vi "GV_YscaleCursorInView.vi"(8 "error in (no error)":errorcluster, 11 "Gviewer in":refnum<class "Gviewer.lvclass">) -> (0 "error out":errorcluster, 3 "Gviewer out":refnum<class "Gviewer.lvclass">)   [LabVIEW 2020, in "Sgraph_lib_V1.lvlib" / "Gviewer.lvclass"]
doc: "Draw cursors and enable identification of a specific trace so it can be selected\nFor use with Y-scale move/delete action"
uses:
  Gviewer.lvclass
  Gviewer.lvclass/Gviewer.ctl
  b6d83b76-addd-4bb4-aca8-673370ce0a1b.vi
  <vilib>/Comparison/Equal/Equal Functor/Equal Functor.lvclass
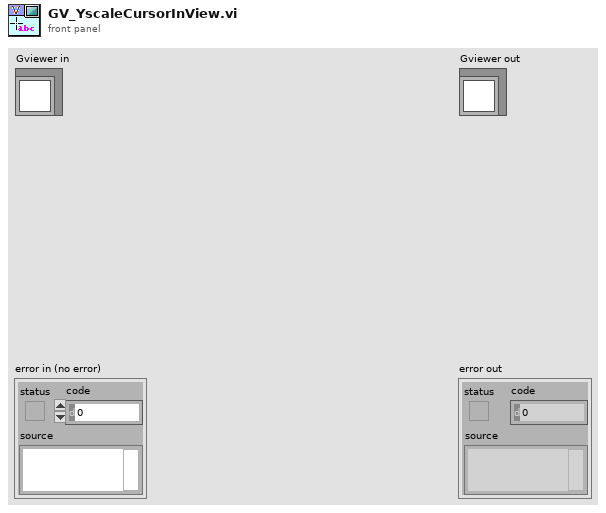
[diagram p1: front panel]
types:
  T1 = typedef "LVPoint32TypeDef.ctl" = cluster{"Horizontal":i32, "Vertical":i32}
  T2 = typedef "LVPositionTypeDef.ctl" = cluster{"Left":i32, "Top":i32}
  T3 = typedef "Sgraph_lib_V1.lvlib/Gviewer.lvclass/YgraphDef.ctl" = cluster{"Plot":i32, "X(%)":dbl}
  T4 = typedef "LVRectTypeDef.ctl" = cluster{"Left":i16, "Top":i16, "Right":i16, "Bottom":i16}
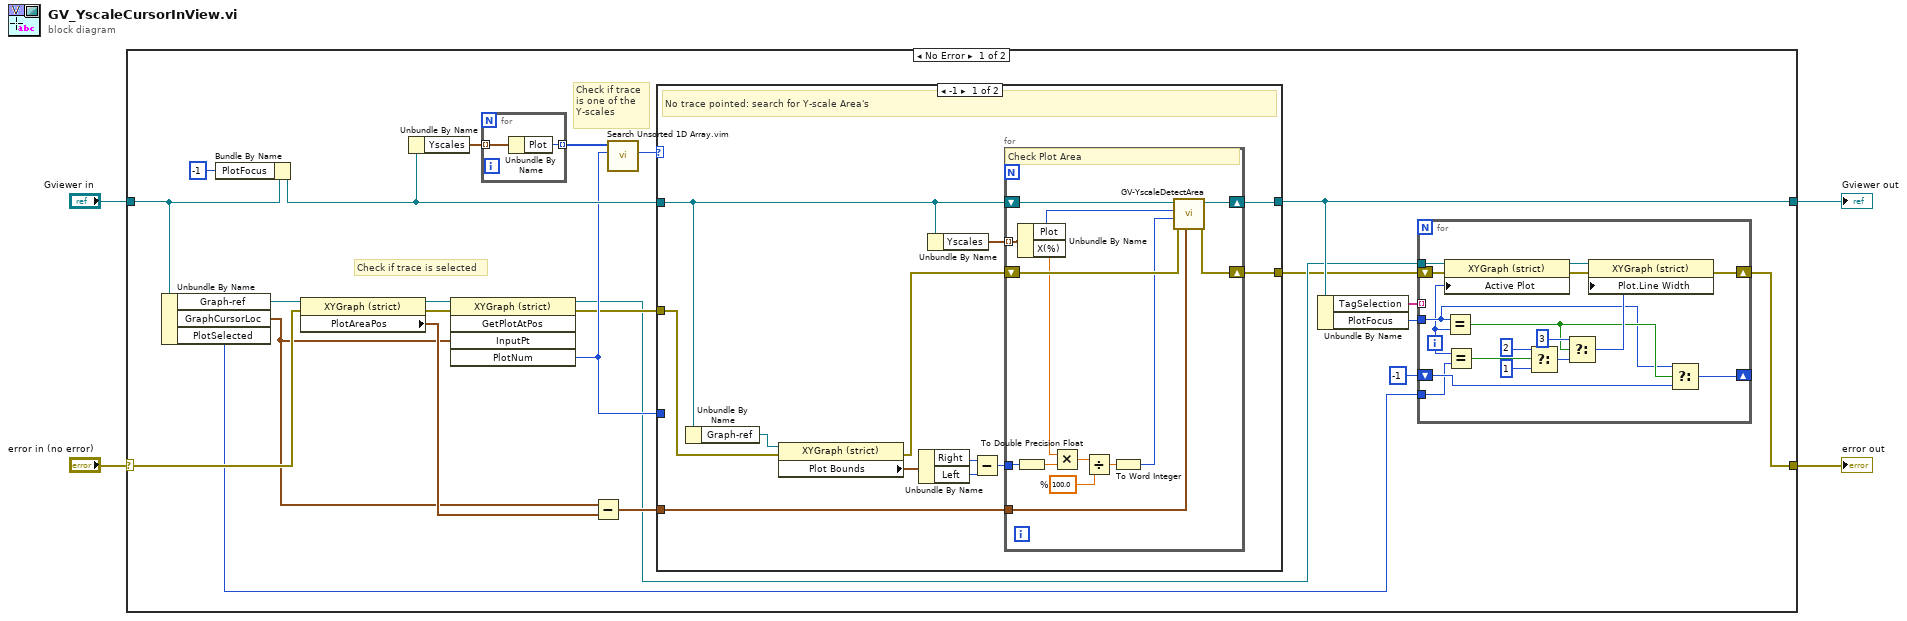
[diagram p0: block diagram]
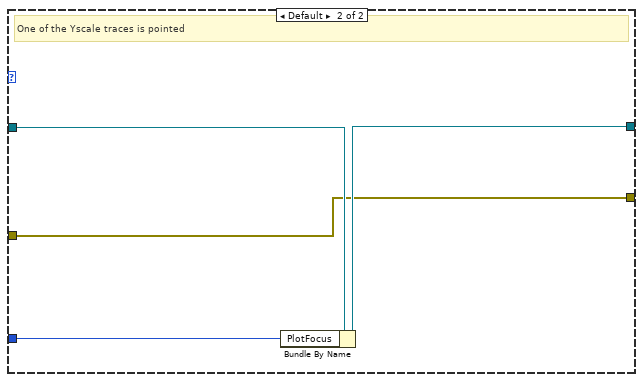
[diagram p2: hidden frame]
diagram:
  n1 = case shown="No Error" "error in (no error)" {
    selector: "error in (no error)" -> [w22 w78]
    tunnel: [w6 w78] -> w3
    tunnel: [w10 w77] -> w1
    tunnel: "Gviewer in" -> [w16 w77]
    frame No Error {
      # "Check if trace\nis one of the\nY-scales"
      # "Check if trace is selected"
      n2 = Unbundle By Name(w16) -> ("Graph-ref"=w24:refnum<vi>, "GraphCursorLoc"=w19:T1, "PlotSelected"=w11:i32)
      n3 = Bundle By Name(cluster=w16, "PlotFocus"=-1) -> (w17:refnum<class "Gviewer.lvclass">)
      n4 = property class="XYGraph (strict)"(reference=w24, error in=w22) -> (reference out=w23:refnum<vi>, error out=w21:errorcluster, "PlotAreaPos"=w20:T2)
      n5 = Unbundle By Name(w17) -> ("Yscales"=w27:T3[])
      n6 = invoke class="XYGraph (strict)" method="GetPlotAtPos"(reference=w23, error in=w21, "InputPt"=w19) -> (reference out=w8:refnum<vi>, error out=w13:errorcluster, "PlotNum"=w14:i32)  [unwired: 2 in, 2 out]
      n7 = for {
        tunnel: w27 -> [w76] mode=indexing
        tunnel: [w75] -> w26 mode=indexing
        n8 = Unbundle By Name(w76) -> ("Plot"=w75:i32)
      }
      n9 = Subtract(x=w19, y=w20) -> (x-y=w18:T1)
      n10 = call "Search Unsorted 1D Array.vim"("element"=w14, "unsorted 1D array"=w26) -> ("index of element"=w25:i32)  [unwired: 9 in]
      n11 = case shown="-1" w25 {
        tunnel: [w49 w74] -> w10
        tunnel: w17 -> [w48 w73]
        tunnel: w14 -> [_ w72]
        tunnel: w13 -> [w52 w71]
        tunnel: [w46 w71] -> w7
        tunnel: w18 -> [w45 _]
        frame -1 {
          # "No trace pointed: search for Y-scale Area's"
          n12 = Unbundle By Name(w48) -> ("Graph-ref"=w53:refnum<vi>)
          n13 = property class="XYGraph (strict)"(reference=w53, error in=w52) -> (error out=w47:errorcluster, "Plot Bounds"=w56:T4)  [unwired: 1 out]
          n14 = Unbundle By Name(w56) -> ("Right"=w54:i16, "Left"=w55:i16)
          n15 = Unbundle By Name(w48) -> ("Yscales"=w51:T3[])
          n16 = Subtract(x=w54, y=w55) -> (x-y=w50:i16)
          n17 = for {
            tunnel: w51 -> [w68] mode=indexing
            shift-right: [w65] -> w46
            shift-left: w47 -> [w66]
            shift-right: [w69] -> w49
            shift-left: w48 -> [w70]
            tunnel: w50 -> [w64]
            tunnel: w45 -> [w57]
            w61 = 100.0  # %
            # "Check Plot Area"
            n18 = To Double Precision Float(number=w64) -> (double precision float=w58:dbl)
            n19 = Unbundle By Name(w68) -> ("Plot"=w67:i32, "X(%)"=w63:dbl)
            n20 = Multiply(x=w63, y=w58) -> (x*y=w62:dbl)
            n21 = Divide(x=w62, y=w61) -> (x/y=w60:dbl)
            n22 = To Word Integer(number=w60) -> (16bit integer=w59:i16)
            n23 = call "GV-YscaleDetectArea.vi"("GraphCursorLoc"=w57, "error in (no error)"=w66, "X-position"=w59, "Plot"=w67, "Gviewer in"=w70) -> ("error out"=w65:errorcluster, "Gviewer out"=w69:refnum<class "Gviewer.lvclass">)  [unwired: 5 in]
          }
        }
        frame Default {
          # "One of the Yscale traces is pointed"
          n24 = Bundle By Name(cluster=w73, "PlotFocus"=w72) -> (w74:refnum<class "Gviewer.lvclass">)
        }
      }
      n25 = Unbundle By Name(w10) -> ("TagSelection"=w5:string[], "PlotFocus"=w9:i32)
      n26 = for {
        tunnel: w9 -> [w34]
        tunnel: w8 -> [w44]
        shift-right: [w38] -> w6
        shift-left: w7 -> [w40]
        shift-right: [w35] -> _
        shift-left: -1 -> [w36]
        tunnel: w11 -> [w31]
        tunnel: w5 -> [_] mode=indexing
        i -> [w32]
        n27 = property class="XYGraph (strict)"(reference=w44, error in=w40, "Active Plot"=w32) -> (reference out=w43:refnum<vi>, error out=w39:errorcluster)
        n28 = Equal?(x=w34, y=w32) -> (x = y?=w37:bool)
        n29 = Equal?(x=w32, y=w31) -> (x = y?=w30:bool)
        n30 = Select(t=u8 2 ("Plot.Line Width"), s=w30, f=u8 1 ("Plot.Line Width")) -> (s? t:f=w33:u8)
        n31 = Select(t=u8 3 ("Plot.Line Width"), s=w37, f=w33) -> (s? t:f=w41:u8)
        n32 = property class="XYGraph (strict)"(reference=w43, error in=w39, "Plot.Line Width"=w41) -> (error out=w38:errorcluster)  [unwired: 1 out]
        n33 = Select(t=w34, s=w37, f=w36) -> (s? t:f=w35:i32)
      }
    }
    frame Error {
    }
  }
  "error out" <- w3
  "Gviewer out" <- w1
